vi "my_tracking.vi"() -> ()   [LabVIEW 2020]
uses:
  <vilib>/Utility/file.llb/Read Delimited Spreadsheet (DBL).vi
  <vilib>/Instr/_visa.llb/VISA Configure Serial Port (Instr).vi
panel:
  in  "VISA resource name":refnum<visa-resource-name>
  out "UTC":dbl
  out "Longtitude":dbl
  out "Latitude":dbl
  out "도(lat)":string
  out "도분초(lat)":string
  out "도(lon)":string
  out "도분초(lon)":string
  out "XYGraph":cluster{"array":dbl[], "array":dbl[]}[](graph)
  out "Satellited Used":string
  out "Fix Position":string
  out "velocity":dbl
  out "String":string
  out "error out":errorcluster
  out "XY graph":cluster{"X":dbl, "Y":dbl}[](graph)
  out "XY DATA":cluster{"X":dbl, "Y":dbl}[](array[cluster])
  out "Clustering graph":T1(graph)
  out "Safe Box Plotting":cluster{dbl[], dbl[]}[](graph)
  out "Box Point Array":cluster{dbl[], dbl[]}[](array[cluster])
  in  "?":enum32{"State", "ETC"}(tab)
  in  "stop":bool
  in  "file path (dialog if empty)":path caption="RDDF"
  out "XY Graph":T2(graph)
  in  "Refresh":bool
  in  "A/M":bool=TRUE
  in  "Serial Name":refnum<visa-resource-name>="COM8"
  out "ERP_Serial_DATA(RAW)":string
  in  "Vel":dbl=4.0 format="%#_13g"
  out "Index(near vehicle)":i32
  out "WP_no.":i32
  out "TM_Y":dbl format="%#_6f"
  out "TM_X":dbl format="%#_6f"
  out "True_Heading":dbl
  out "x_lat_path":dbl[](array[numeric])
  out "y_long_path":dbl[](array[numeric])
  out "vel. path":dbl[](array[numeric])
  out "Path_Vel_arr":dbl[](array[numeric])
  out "Path_long_arr":dbl[](array[numeric])
  out "Path_lat_arr":dbl[](array[numeric])
  out "ERP_Receive":T3
  out "Steer_CMD(Deg)":dbl
  out "CMD_2_ERP":T4
  out "Brake":u8
  out "Tracking_Error(m)":dbl
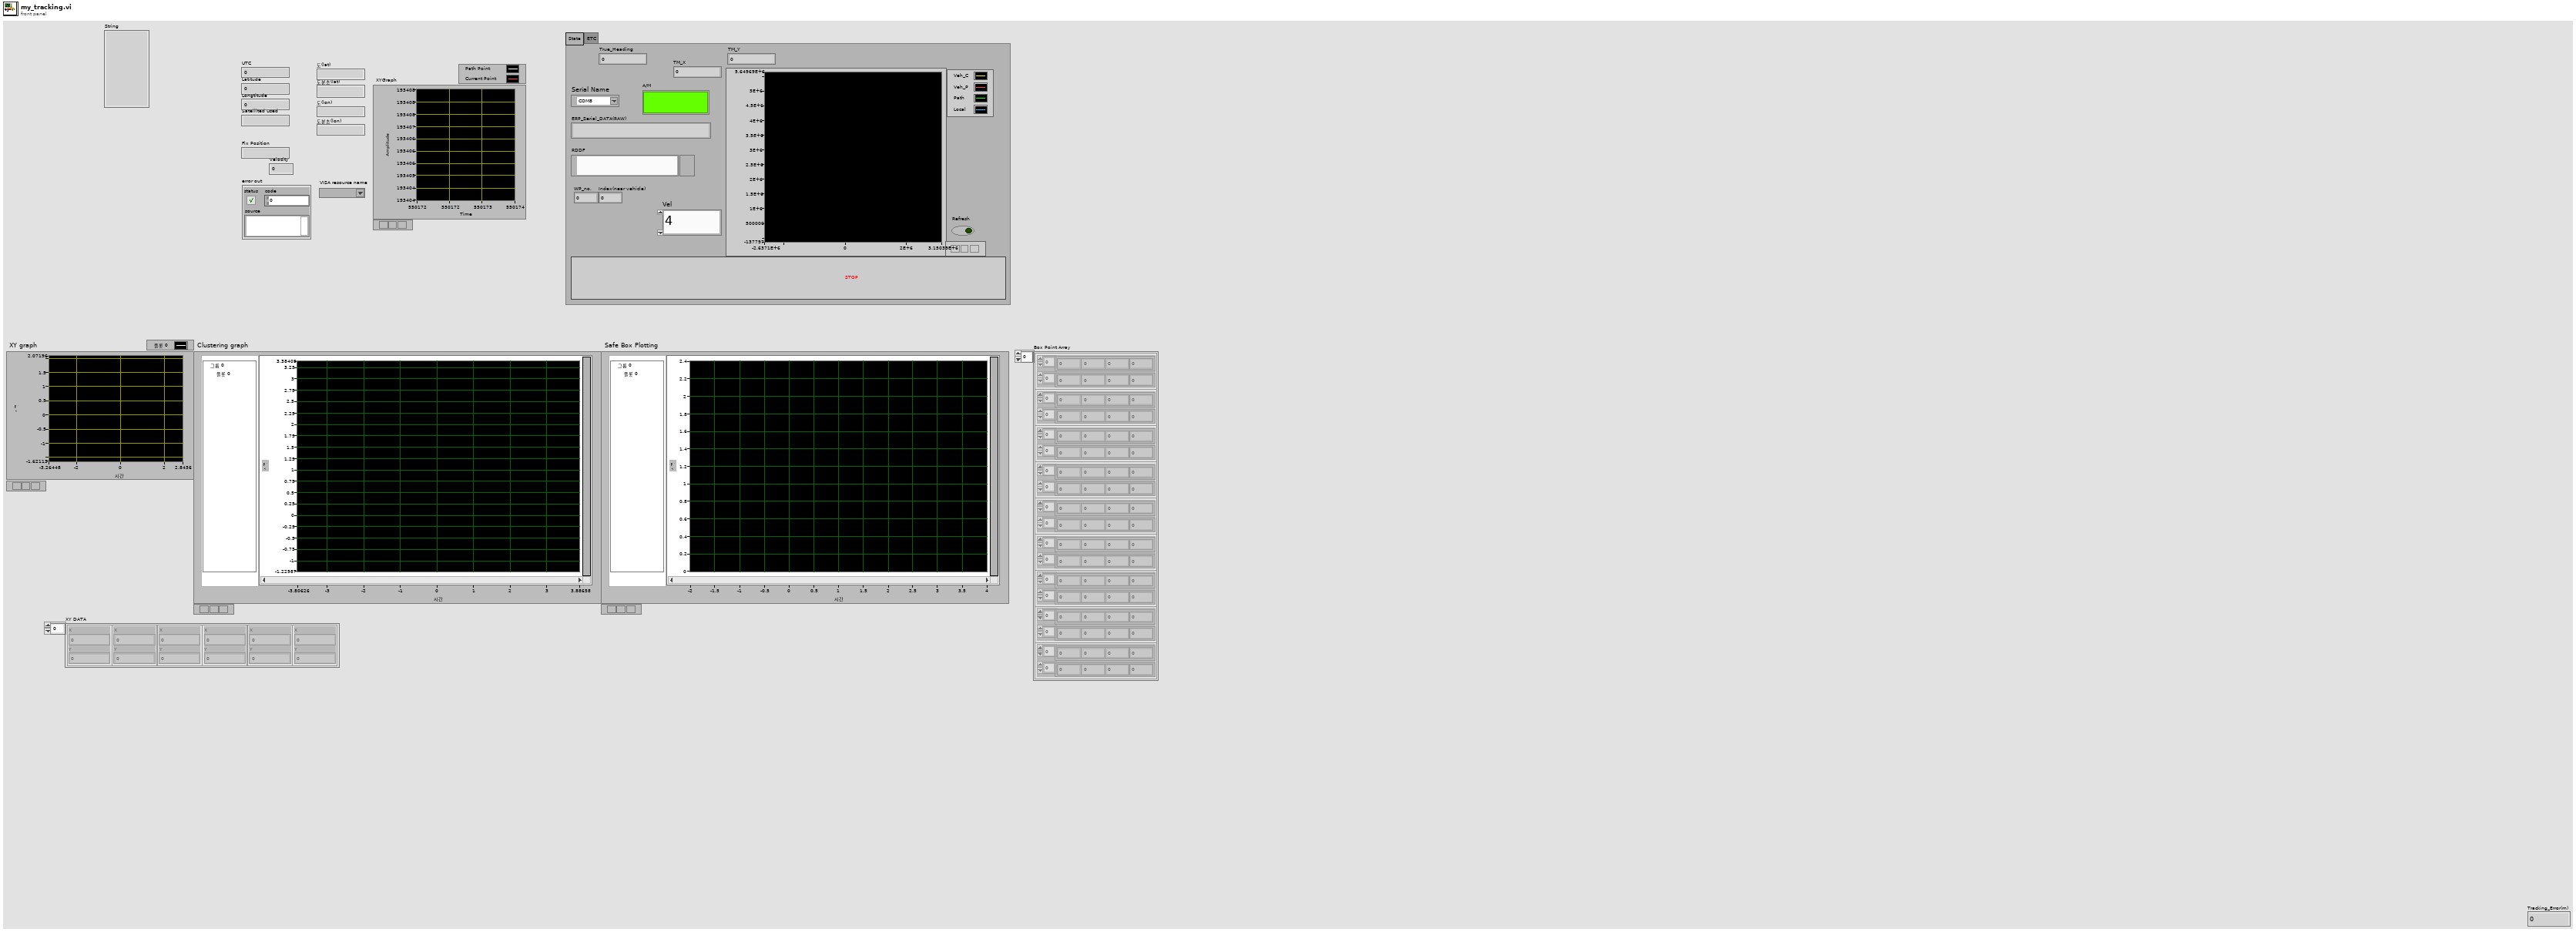
[diagram p1: front panel]
types:
  T1 = cluster{"최종 클러스터링 배열":cluster{"X":dbl, "Y":dbl}[]}[]
  T2 = cluster{"y_long_path":dbl[], "x_lat_path":dbl[]}[]
  T3 = cluster{"AorM":u8, "E-Stop":u8, "F_B":u8, "Speed":u16, "Steer":i16, "Brake":u8, "Encoder":u8, "Encoder 2":u8, "Encoder 3":u8, "Encoder 4":u8, "ALIVE":u8, "ETX_0":u8, "ETX_0 2":u8}
  T4 = cluster{"F/B":u8, "Speed":u16, "Steer":i16, "A/M":u8, "Brake":u8}
  T5 = cluster{"S":u8, "T":u8, "X":u8, "AorM":u8, "E-Stop":u8, "F_B":u8, "Speed":u16, "Steer":i16, "Brake":u8, "ALIVE":u8, "ETX_0":u8, "ETX_0 2":u8}
  T6 = cluster{"Path_long_arr":dbl[], "Path_lat_arr":dbl[]}
  T7 = cluster{"Path_long_arr":dbl[], "Path_lat_arr":dbl[]}[]
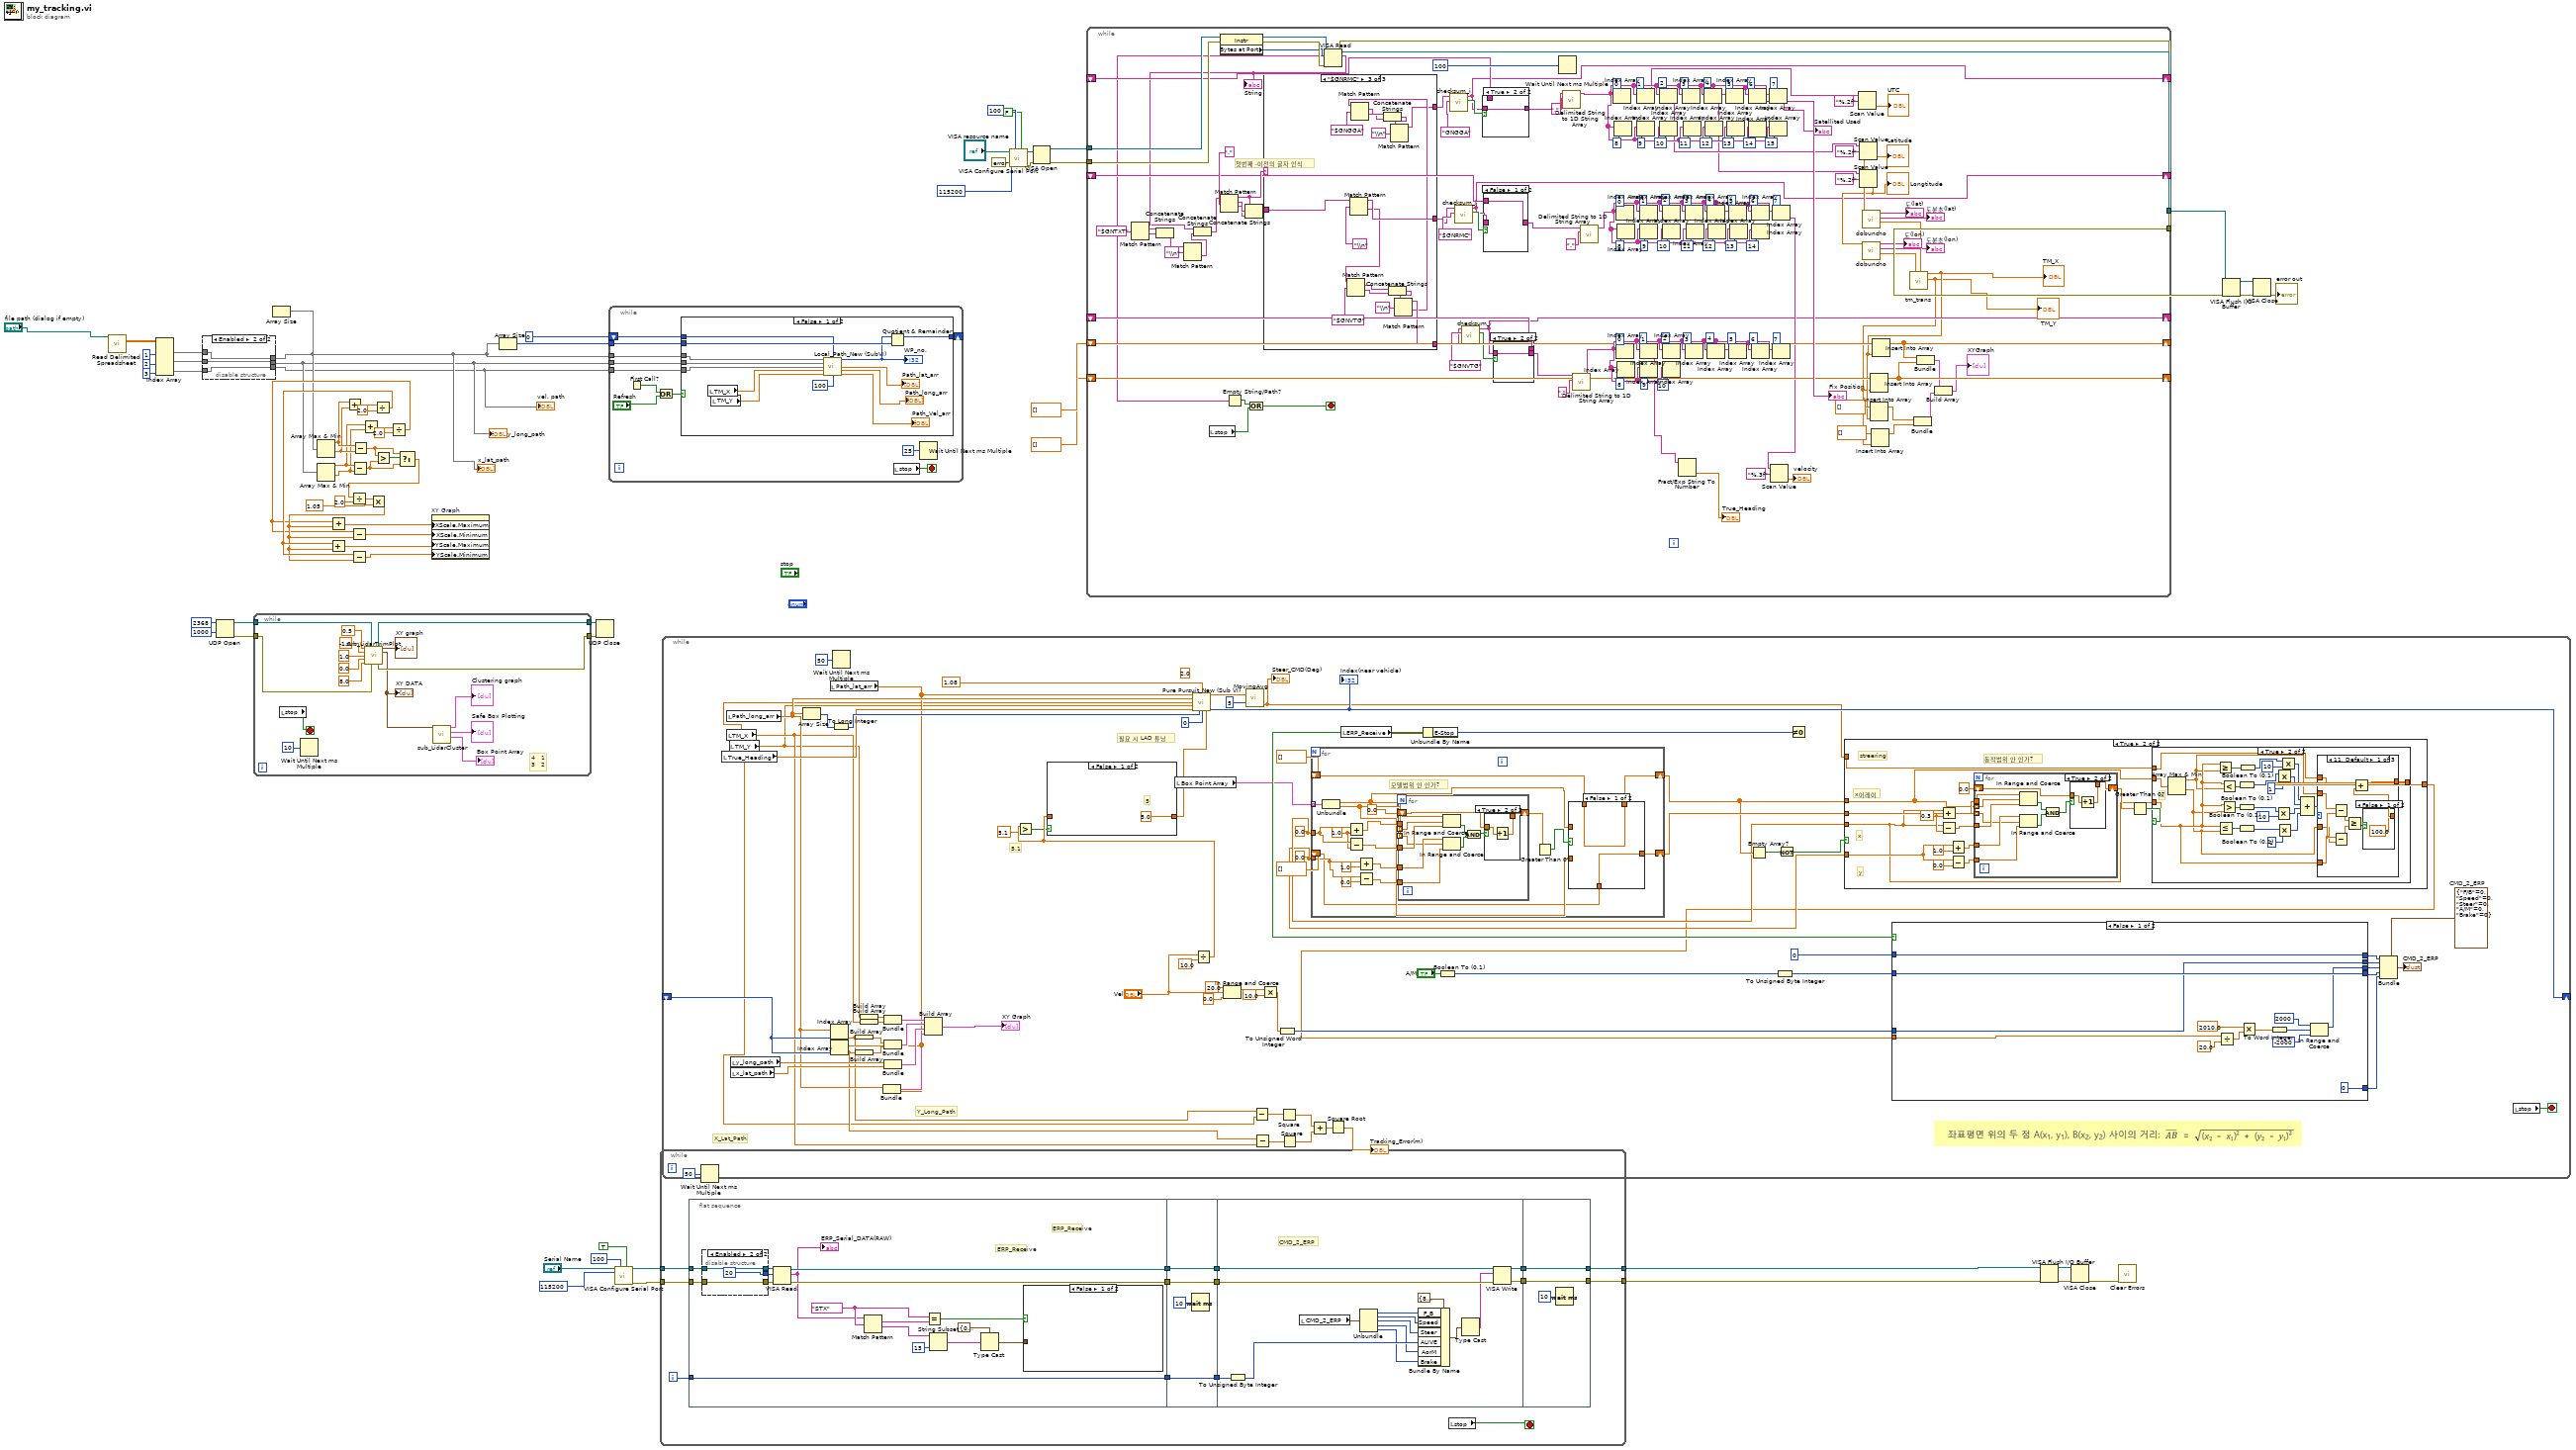
[diagram p0: block diagram]
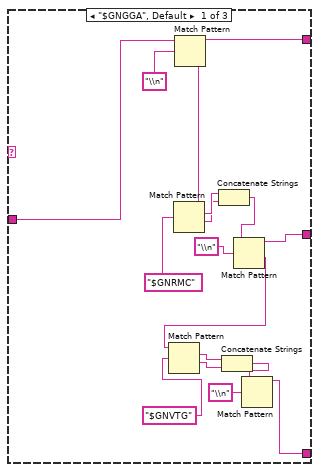
[diagram p5: hidden frame]
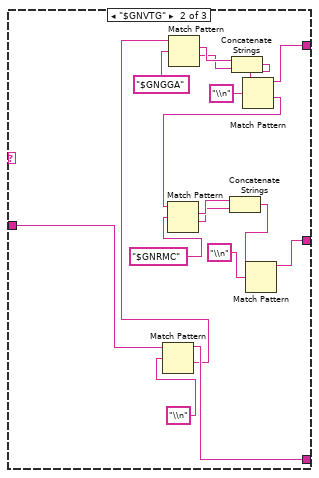
[diagram p6: hidden frame]
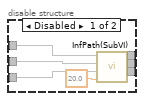
[diagram p7: hidden frame]
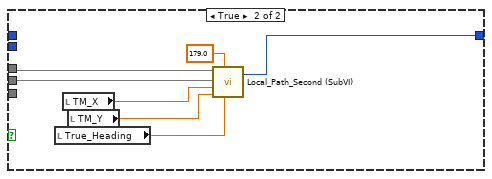
[diagram p8: hidden frame]
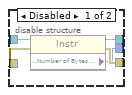
[diagram p9: hidden frame]
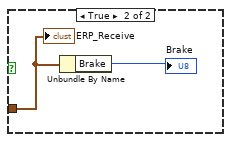
[diagram p10: hidden frame]
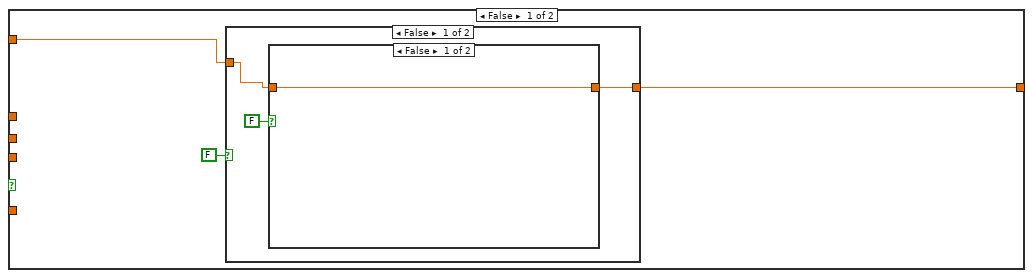
[diagram p11: hidden frame]
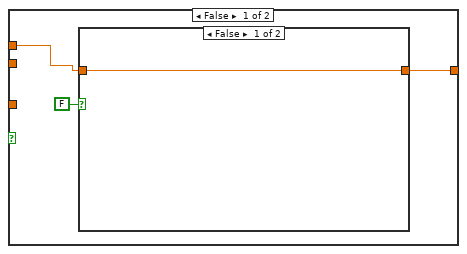
[diagram p15: hidden frame]
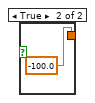
[diagram p17: hidden frame]
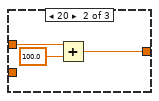
[diagram p18: hidden frame]
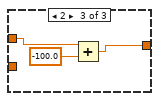
[diagram p19: hidden frame]
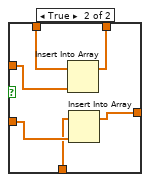
[diagram p20: hidden frame]
diagram:
  n1 = call-poly <vilib>:"Read Delimited Spreadsheet.vi"("file path (dialog if empty)"="file path (dialog if empty)") -> ("all rows"=w29:dbl[][])  [unwired: 9 in, 5 out]
  n2 = Index Array(array=w29, index (col) #1=1 ("비활성화된 인덱스 (열)"), index (col) #2=2 ("인덱스 (열)"), index (col) #3=3 ("인덱스 (열)")) -> (element #1=w54:dbl[], element #2=w53:dbl[], element #3=w52:dbl[])  [unwired: 3 in]
  n3 = disable-structure shown="Enabled" {
    disable-tunnel: w54 -> [w75 w78]
    disable-tunnel: w53 -> [w74 w77]
    disable-tunnel: w52 -> [w73 w76]
    disable-tunnel: [w72 w77] -> w18
    disable-tunnel: [w71 w76] -> w17
    disable-tunnel: [w70 w78] -> w19
    frame Disabled {
      n4 = call "InfPath(SubVI).vi"("Mod dist."=20.0, "vel."=w73, "y_long"=w74, "x_lat"=w75) -> ("vel. path"=w71:dbl[], "y_long_path"=w72:dbl[], "x_lat_path"=w70:dbl[])  [unwired: 1 out]
    }
    frame Enabled {
    }
  }
  "vel. path" <- w17
  "x_lat_path" <- w19
  "y_long_path" <- w18
  n5 = UDP Open(9:1000 ("타임아웃 ms (25000)"), 11:u16 2368 ("포트")) -> (port=w23:refnum<k16>, 0:w24:errorcluster)  [unwired: 3 in, 1 out]
  n6 = while {
    tunnel: w23 -> [w88]
    tunnel: w24 -> [w87]
    tunnel: [w86] -> w22
    tunnel: [w85] -> w21
    stop <- w79 stop-if-true
    # "4   1\n3   2"
    n7 = local read "stop"() -> (w79:bool)
    n8 = Wait Until Next ms Multiple(millisecond multiple=u32 10 ("ms 배수")) -> ()  [unwired: 1 out]
    n9 = call "sub_LidarTrimPlot.vi"("R_min"=0.5, "UDP 네트워크 연결 입력"=w88, "x-"=-1.0, "x+"=1.0, "y-"=0.0, "y+"=8.0, "에러 입력(에러 없음)"=w87) -> ("UDP 네트워크 연결 출력"=w86:refnum<k16>, "Point Cloud Plotting"=→"XY graph":cluster{"X":dbl, "Y":dbl}[], "trim XY DATA"=w83:cluster{"X":dbl, "Y":dbl}[], "에러 출력"=w85:errorcluster)  [unwired: 5 in]
    "XY DATA" <- w83
    n10 = call "sub_LidarCluster.vi"("XY DATA"=w83) -> ("Box Point Array"=→"Box Point Array":cluster{dbl[], dbl[]}[], "Safe Box Plotting"=→"Safe Box Plotting":cluster{dbl[], dbl[]}[], "Cluster Plotting"=→"Clustering graph":T1)  [unwired: 8 in]
  }
  n11 = Array Size(array=w19) -> ()  [unwired: 1 out]
  n12 = Array Max & Min(array=w18) -> (max value=w40:dbl, min value=w39:dbl)  [unwired: 2 out]
  n13 = Array Max & Min(array=w19) -> (max value=w46:dbl, min value=w45:dbl)  [unwired: 2 out]
  n14 = Add(x=w46, y=w45) -> (x+y=w43:dbl)
  n15 = Subtract(x=w40, y=w39) -> (x-y=w49:dbl)
  n16 = Subtract(x=w46, y=w45) -> (x-y=w50:dbl)
  n17 = Add(x=w40, y=w39) -> (x+y=w42:dbl)
  n18 = Divide(x=w43, y=2.0) -> (x/y=w36:dbl)
  n19 = Greater?(x=w50, y=w49) -> (0:w51:bool)
  n20 = Divide(x=w42, y=2.0) -> (x/y=w28:dbl)
  n21 = Select(t=w50, s=w51, f=w49) -> (s? t:f=w47:dbl)
  n22 = Divide(x=w47, y=2.0) -> (x/y=w38:dbl)
  n23 = Multiply(x=w38, y=1.05) -> (x*y=w35:dbl)
  n24 = Add(x=w36, y=w35) -> (x+y=w33:dbl)
  n25 = Add(x=w28, y=w35) -> (x+y=w31:dbl)
  n26 = Subtract(x=w28, y=w35) -> (x-y=w32:dbl)
  n27 = Subtract(x=w36, y=w35) -> (x-y=w34:dbl)
  n28 = property on="XY Graph" class="XYGraph (strict)"("XScale.Maximum"=w31, "XScale.Minimum"=w32, "YScale.Maximum"=w33, "YScale.Minimum"=w34) -> ()  [unwired: 2 in, 2 out]
  n29 = Array Size(array=w19) -> (size(s)=w30:i32)
  n30 = UDP Close(connection ID=w22, 8:w21) -> ()  [unwired: 2 out]
  n31 = while {
    tunnel: w19 -> [w104]
    tunnel: w18 -> [w103]
    tunnel: w17 -> [w101]
    tunnel: w30 -> [w100]
    shift-right: [w99] -> _
    shift-left: 0 ("Index0") -> [w102]
    stop <- w105 stop-if-true
    n32 = First Call?() -> (First Call?: T/F=w97:bool)
    n33 = Or(x=w97, y="Refresh") -> (x .or. y?=w98:bool)
    n34 = case shown="False" w98 {
      tunnel: w104 -> [w110 w125]
      tunnel: w103 -> [w112 w124]
      tunnel: w102 -> [w113 _]
      tunnel: w101 -> [w111 _]
      tunnel: w100 -> [w117 _]
      tunnel: [w118 w119] -> w99
      frame False {
        n35 = local read "TM_X"() -> (w116:dbl)
        n36 = local read "TM_Y"() -> (w115:dbl)
        n37 = call "Local_Path_New (SubVI).vi"("x_lat_arr"=w110, "WP no_pre"=w113, "y_long_arr"=w112, "vel_arr"=w111, "x_lat_c"=w116, "y_long_c"=w115, "# of pnt"=100) -> ("INDEX(Near Point)"=w107:i32, "Lat(Local)"=→"Path_lat_arr":dbl[], "Long(Local)"=→"Path_long_arr":dbl[], "Vel(Local)"=→"Path_Vel_arr":dbl[])  [unwired: 5 in]
        "WP_no." <- w107
        n38 = Quotient & Remainder(x=w107, y=w117) -> (x-y*floor(x/y)=w118:i32)  [unwired: 1 out]
      }
      frame True {
        n39 = local read "True_Heading"() -> (w121:dbl)
        n40 = local read "TM_X"() -> (w123:dbl)
        n41 = local read "TM_Y"() -> (w122:dbl)
        n42 = call "Local_Path_Second (SubVI).vi"("heading_deg"=w121, "heading_limit"=179.0, "y_long"=w122, "x_lat"=w123, "Y_long_path"=w124, "X_lat_path"=w125) -> ("Index(near vehicle)"=w119:i32)  [unwired: 1 out]
      }
    }
    n43 = local read "stop"() -> (w105:bool)
    n44 = Wait Until Next ms Multiple(millisecond multiple=u32 25) -> ()  [unwired: 1 out]
  }
  n45 = call-poly "VISA Configure Serial Port"("VISA resource name"="Serial Name", "timeout (10sec)"=u32 100, "Enable Termination\nChar (T)"=TRUE ("Enable Termination\nChar (T)"), "baud rate (9600)"=u32 115200) -> ("VISA resource name out"=w60:refnum<visa-resource-name>, "error out"=w59:errorcluster)  [unwired: 10 in]
  n46 = while {
    tunnel: w60 -> [w139]
    tunnel: w59 -> [w138]
    tunnel: [w136] -> w62
    tunnel: [w135] -> w61
    i -> [w137]
    stop <- w128 stop-if-true
    n47 = flat-sequence {
      tunnel: w139 -> [w157]
      tunnel: w138 -> [w156]
      tunnel: [w155] -> w134
      tunnel: [w154] -> w132
      tunnel: w137 -> [w153]
      tunnel: [w153] -> w130
      tunnel: w134 -> [w171]
      tunnel: [w171] -> w133
      tunnel: w132 -> [w170]
      tunnel: [w170] -> w131
      tunnel: w130 -> [w169]
      tunnel: [w169] -> w129
      tunnel: w133 -> [w184]
      tunnel: w131 -> [w183]
      tunnel: w129 -> [w181]
      tunnel: [w180] -> w127
      tunnel: [w179] -> w126
      tunnel: [w188] -> w135
      tunnel: [w189] -> w136
      tunnel: w127 -> [w189]
      tunnel: w126 -> [w188]
      frame #0 {
        w147 = "STX" ("검색 문자열/문자 (-)")
        # "ERP_Receive"
        # "ERP_Receive"
        n48 = disable-structure shown="Enabled" {
          disable-tunnel: w157 -> [w162 w164]
          disable-tunnel: w156 -> [w161 w165]
          disable-tunnel: [w160 w165] -> w152
          disable-tunnel: [w159 u32 20 ("timeout (10sec)")] -> w151
          disable-tunnel: [w158 w164] -> w150
          frame Disabled {
            n49 = property class="Instr"(reference=w162, error in=w161) -> (reference out=w158:refnum<visa-resource-name>, error out=w160:errorcluster, "Serial Settings:Number of Bytes at Serial Port"=w159:u32)
          }
          frame Enabled {
          }
        }
        n50 = VISA Read(VISA resource name=w150, byte count=w151, error in (no error)=w152) -> (VISA resource name out=w155:refnum<visa-resource-name>, read buffer=w145:string, error out=w154:errorcluster)  [unwired: 1 out]
        "ERP_Serial_DATA(RAW)" <- w145
        n51 = Match Pattern(string=w145, regular expression=w147) -> (match substring=w146:string, after substring=w149:string)  [unwired: 1 in, 2 out]
        n52 = Equal?(x=w147, y=w146) -> (x = y?=w144:bool)
        n53 = String Subset(string=w149, length (rest)=15 ("길이(나머지)")) -> (substring=w143:string)  [unwired: 1 in]
        n54 = Type Cast(type=T3 {"AorM"=0, "E-Stop"=0, "F_B"=0, "Speed"=0, "Steer"=0, "Brake"=0, "Encoder"=0, "Encoder 2"=0, "Encoder 3"=0, "Encoder 4"=0, "ALIVE"=0, "ETX_0"=13, "ETX_0 2"=10}, x=w143) -> (*(type *) &x=w142:T3)
        n55 = case shown="False" w144 {
          tunnel: w142 -> [_ w167]
          frame False {
          }
          frame True {
            n56 = Unbundle By Name(w167) -> ("Brake"=→"Brake":u8)
            "ERP_Receive" <- w167
          }
        }
      }
      frame #1 {
        n57 = Wait (ms)(milliseconds to wait=u32 10 ("대기 시간(ms)")) -> ()  [unwired: 1 out]
      }
      frame #2 {
        # "CMD_2_ERP"
        n58 = To Unsigned Byte Integer(number=w181) -> (unsigned 8bit integer=w186:u8)
        n59 = local read "CMD_2_ERP"() -> (w173:T4)
        n60 = Unbundle(w173) -> ("F/B"=w178:u8, "Speed"=w177:u16, "Steer"=w176:i16, "A/M"=w174:u8, "Brake"=w172:u8)
        n61 = Bundle By Name(cluster=T5 {"S"=83, "T"=84, "X"=88, "AorM"=0, "E-Stop"=0, "F_B"=0, "Speed"=0, "Steer"=0, "Brake"=0, "ALIVE"=0, "ETX_0"=13, "ETX_0 2"=10}, "F_B"=w178, "Speed"=w177, "Steer"=w176, "ALIVE"=w186, "AorM"=w174, "Brake"=w172) -> (w185:T5)
        n62 = Type Cast(x=w185) -> (*(type *) &x=w182:string)  [unwired: 1 in]
        n63 = VISA Write(VISA resource name=w184, write buffer=w182, error in (no error)=w183) -> (VISA resource name out=w180:refnum<visa-resource-name>, error out=w179:errorcluster)  [unwired: 1 out]
      }
      frame #3 {
        n64 = Wait (ms)(milliseconds to wait=u32 10 ("대기 시간(ms)")) -> ()  [unwired: 1 out]
      }
    }
    n65 = Wait Until Next ms Multiple(millisecond multiple=u32 50 ("ms 배수")) -> ()  [unwired: 1 out]
    n66 = local read "stop"() -> (w128:bool)
  }
  n67 = while {
    shift-right: [w247] -> _
    shift-left: _ -> [w244]
    stop <- w253 stop-if-true
    w192 = 0.0 ("TM_Y")
    w193 = 0.0 ("TM_X")
    w219 = T4 {"F/B"=0, "Speed"=0, "Steer"=0, "A/M"=0, "Brake"=0}  # CMD_2_ERP
    (unwired) 2.0 ("L")
    # "5.1"
    # "X_Lat_Path"
    # "Y_Long_Path"
    # "필요 시 LAD 튜닝"
    n68 = local read "True_Heading"() -> (w240:dbl)
    n69 = local read "Path_long_arr"() -> (w216:dbl[])
    n70 = local read "TM_X"() -> (w201:dbl)
    n71 = local read "TM_Y"() -> (w200:dbl)
    n72 = local read "y_long_path"() -> (w224:dbl[])
    n73 = local read "x_lat_path"() -> (w223:dbl[])
    n74 = Array Size(array=w216) -> (size(s)=w248:i32)
    n75 = local read "Path_lat_arr"() -> (w215:dbl[])
    n76 = Index Array(array=w216, index=w244) -> (element=w206:dbl)
    n77 = Index Array(array=w215, index=w244) -> (element=w205:dbl)
    n78 = Wait Until Next ms Multiple(millisecond multiple=u32 50 ("ms 배수")) -> ()  [unwired: 1 out]
    n79 = To Long Integer(number=w248) -> (32bit integer=w246:i32)
    n80 = Build Array(w206) -> (w255:dbl[])
    n81 = Build Array(w205) -> (w254:dbl[])
    n82 = Build Array(w200) -> (w257:dbl[])
    n83 = Build Array(w201) -> (w256:dbl[])
    n84 = Bundle("Path_long_arr"=w216, "Path_lat_arr"=w215) -> (w236:T6)  [unwired: 1 in]
    n85 = Bundle(w257, w256) -> (w242:cluster{dbl[], dbl[]})  [unwired: 1 in]
    n86 = Bundle(w255, w254) -> (w241:cluster{dbl[], dbl[]})  [unwired: 1 in]
    n87 = Bundle("y_long_path"=w224, "x_lat_path"=w223) -> (w243:cluster{"y_long_path":dbl[], "x_lat_path":dbl[]})  [unwired: 1 in]
    n88 = Build Array(w242, w241, w243, w236) -> (→"XY Graph":T7)
    n89 = local read "Box Point Array"() -> (w202:cluster{dbl[], dbl[]}[])
    n90 = Divide(x="Vel", y=10.0) -> (x/y=w237:dbl)
    n91 = Greater?(x=w237, y=5.1) -> (0:w204:bool)
    n92 = case shown="False" w204 {
      tunnel: w237 -> [_ w388]
      tunnel: [5.0 w387] -> w239
      frame False {
        # "5"
      }
      frame True {
        w389 = 3.7978021978021976  # intercept
        w391 = 0.23736263736263735  # slope
        n93 = Multiply(x=w391, y=w388) -> (x*y=w390:dbl)
        n94 = Add(x=w390, y=w389) -> (x+y=w387:dbl)
      }
    }
    n95 = call "Pure Pursuit_New (Sub VI).vi"("x_lat_path"=w215, "L"=1.08, "y_long_path"=w216, "X_Current"=w201, "Y_Current"=w200, "Heading_Current"=w240, "#pnt"=w246, "WP no_pre"=0, "LAD"=w239) -> ("Steer_CMD(Deg)"=w214:dbl, "Index(near vehicle)"=w247:i32)  [unwired: 5 in]
    "Index(near vehicle)" <- w247
    n96 = In Range and Coerce(upper limit=20.0 ("상위 리미트"), x="Vel", lower limit=0.0 ("하위 리미트")) -> (coerced(x)=w228:dbl)  [unwired: 1 out]
    n97 = call "MovingAvg.vi"("입력"=w214, "이동평균을 구할 자료의 개수"=u16 5) -> ("이동평균"=w191:dbl)  [unwired: 2 out]
    "Steer_CMD(Deg)" <- w191
    n98 = Subtract(x=w206, y=w200) -> (x-y=w211:dbl)
    n99 = Subtract(x=w205, y=w201) -> (x-y=w210:dbl)
    n100 = Multiply(x=w228, y=10.0) -> (x*y=w226:dbl)
    n101 = To Unsigned Word Integer(number=w226) -> (unsigned 16bit integer=w232:u16)
    n102 = Square(x=w211) -> (x^2=w209:dbl)
    n103 = Square(x=w210) -> (x^2=w208:dbl)
    n104 = for {
      tunnel: w202 -> [w363] mode=indexing
      tunnel: w193 -> [w356]
      tunnel: w192 -> [w354]
      shift-right: [w348] -> w196
      shift-left: dbl[] [] -> [w349]
      shift-right: [w346] -> w197
      shift-left: dbl[] [] -> [w345]
      w355 = 1.0 ("y")
      # "모델범위 안 인가?"
      n105 = Unbundle(w363) -> (w350:dbl[], w347:dbl[])
      n106 = Add(x=w356, y=w355) -> (x+y=w360:dbl)
      n107 = Subtract(x=w356, y=w355) -> (x-y=w359:dbl)
      n108 = Add(x=w354, y=1.0) -> (x+y=w358:dbl)
      n109 = Subtract(x=w354, y=0.0) -> (x-y=w357:dbl)
      n110 = for {
        tunnel: w350 -> [w380] mode=indexing
        tunnel: w347 -> [w377] mode=indexing
        tunnel: w360 -> [w382]
        tunnel: w359 -> [w381]
        tunnel: w358 -> [w379]
        tunnel: w357 -> [w378]
        shift-right: [w372] -> w353
        shift-left: 0.0 -> [w373]
        n111 = In Range and Coerce(upper limit=w382, x=w380, lower limit=w381) -> (In Range?=w376:bool)  [unwired: 1 out]
        n112 = In Range and Coerce(upper limit=w379, x=w377, lower limit=w378) -> (In Range?=w375:bool)  [unwired: 1 out]
        n113 = And(x=w376, y=w375) -> (x .and. y?=w374:bool)
        n114 = case shown="True" w374 {
          tunnel: w373 -> [w383 w385]
          tunnel: [w383 w384] -> w372
          frame False {
          }
          frame True {
            n115 = Increment(x=w385) -> (x+1=w384:dbl)
          }
        }
      }
      n116 = Greater Than 0?(x=w353) -> (x > 0?=w351:bool)
      n117 = case shown="False" w351 {
        tunnel: w350 -> [_ w371]
        tunnel: w349 -> [w365 w370]
        tunnel: [w365 w369] -> w348
        tunnel: w347 -> [_ w368]
        tunnel: [w364 w367] -> w346
        tunnel: w345 -> [w364 w366]
        frame False {
        }
        frame True {
          n118 = Insert Into Array(array=w370, new element=w371) -> (w369:dbl[])  [unwired: 1 in]
          n119 = Insert Into Array(array=w366, new element=w368) -> (w367:dbl[])  [unwired: 1 in]
        }
      }
    }
    n120 = Add(x=w209, y=w208) -> (x+y=w207:dbl)
    n121 = Square Root(x=w207) -> (sqrt(x)=→"Tracking_Error(m)":dbl)
    n122 = local read "ERP_Receive"() -> (w250:T3)
    n123 = Unbundle By Name(w250) -> ("E-Stop"=w251:u8)
    n124 = Boolean To (0,1)(Boolean="A/M") -> (0, 1=w235:i16)
    n125 = Empty Array?(array=w196) -> (empty?=w195:bool)
    n126 = To Unsigned Byte Integer(number=w235) -> (unsigned 8bit integer=w217:u8)
    n127 = Not(x=w195) -> (.not. x?=w194:bool)
    n128 = Not Equal To 0?(x=w251) -> (x != 0?=w231:bool)
    n129 = case shown="True" w194 {
      tunnel: w191 -> [w263 w285]
      tunnel: [w262 w284] -> w190
      tunnel: w196 -> [_ w270]
      tunnel: w197 -> [_ w283]
      tunnel: w193 -> [_ w271]
      tunnel: w192 -> [_ w279]
      frame False {
        n130 = case shown="False" FALSE {
          tunnel: w263 -> [w266 w269]
          tunnel: [w265 w269] -> w262
          frame False {
            n131 = case shown="False" FALSE {
              tunnel: w266 -> [w267 w268]
              tunnel: [w267 w268] -> w265
              frame False {
              }
              frame True {
              }
            }
          }
          frame True {
          }
        }
      }
      frame True {
        w280 = 0.3 ("y")
        # "y"
        # "x"
        # "streering"
        # "x어레이"
        # "동작범위 안 인가?"
        n132 = Add(x=w271, y=w280) -> (x+y=w278:dbl)
        n133 = Subtract(x=w271, y=w280) -> (x-y=w277:dbl)
        n134 = Add(x=w279, y=1.0) -> (x+y=w276:dbl)
        n135 = Subtract(x=w279, y=0.0) -> (x-y=w275:dbl)
        n136 = for {
          tunnel: w270 -> [w294] mode=indexing
          tunnel: w283 -> [w291] mode=indexing
          tunnel: w278 -> [w296]
          tunnel: w277 -> [w295]
          tunnel: w276 -> [w293]
          tunnel: w275 -> [w292]
          shift-right: [w288] -> w273
          shift-left: 0.0 -> [w287]
          n137 = In Range and Coerce(upper limit=w296, x=w294, lower limit=w295) -> (In Range?=w290:bool)  [unwired: 1 out]
          n138 = In Range and Coerce(upper limit=w293, x=w291, lower limit=w292) -> (In Range?=w289:bool)  [unwired: 1 out]
          n139 = And(x=w290, y=w289) -> (x .and. y?=w286:bool)
          n140 = case shown="True" w286 {
            tunnel: w287 -> [w297 w299]
            tunnel: [w297 w298] -> w288
            frame False {
            }
            frame True {
              n141 = Increment(x=w299) -> (x+1=w298:dbl)
            }
          }
        }
        n142 = Greater Than 0?(x=w273) -> (x > 0?=w272:bool)
        n143 = case shown="True" w272 {
          tunnel: w285 -> [w302 w310]
          tunnel: [w301 w309] -> w284
          tunnel: w271 -> [_ w308]
          tunnel: w270 -> [_ w307]
          frame False {
            n144 = case shown="False" FALSE {
              tunnel: w302 -> [w303 w304]
              tunnel: [w303 w304] -> w301
              frame False {
              }
              frame True {
              }
            }
          }
          frame True {
            # "x"
            n145 = Array Max & Min(array=w307) -> (max value=w306:dbl, min value=w305:dbl)  [unwired: 2 out]
            n146 = Greater Or Equal?(x=w308, y=w306) -> (x >= y?=w327:bool)
            n147 = Less Or Equal?(x=w308, y=w305) -> (x <= y?=w326:bool)
            n148 = Less?(x=w308, y=w306) -> (x < y?=w312:bool)
            n149 = Greater?(x=w308, y=w305) -> (0:w311:bool)
            n150 = Boolean To (0,1)(Boolean=w312) -> (0, 1=w319:i16)
            n151 = Boolean To (0,1)(Boolean=w311) -> (0, 1=w321:i16)
            n152 = Boolean To (0,1)(Boolean=w326) -> (0, 1=w320:i16)
            n153 = Boolean To (0,1)(Boolean=w327) -> (0, 1=w318:i16)
            n154 = Multiply(x=w321, y=i16 10) -> (x*y=w315:i16)
            n155 = Multiply(x=w319, y=i16 1) -> (x*y=w316:i16)
            n156 = Multiply(x=w320, y=i16 1) -> (x*y=w314:i16)
            n157 = Multiply(x=w318, y=i16 10) -> (x*y=w317:i16)
            n158 = Compound Arithmetic op=ADD(w317, w316, w315, w314) -> (w313:i16)
            n159 = case shown="11, Default" w313 {
              tunnel: w310 -> [w330 w341 w342]
              tunnel: [w328 w339 w343] -> w309
              tunnel: w306 -> [w335 _ _]
              tunnel: w305 -> [w334 _ _]
              tunnel: w308 -> [w336 _ _]
              frame 11, Default {
                n160 = Subtract(x=w335, y=w336) -> (x-y=w333:dbl)
                n161 = Subtract(x=w336, y=w334) -> (x-y=w332:dbl)
                n162 = Greater Or Equal?(x=w333, y=w332) -> (x >= y?=w331:bool)
                n163 = case shown="False" w331 {
                  tunnel: [100.0 -100.0] -> w329
                  frame False {
                  }
                  frame True {
                  }
                }
                n164 = Add(x=w330, y=w329) -> (x+y=w328:dbl)
              }
              frame 20 {
                n165 = Add(x=w341, y=100.0) -> (x+y=w339:dbl)
              }
              frame 2 {
                n166 = Add(x=w342, y=-100.0) -> (x+y=w343:dbl)
              }
            }
          }
        }
      }
    }
    n167 = case shown="False" w231 {
      tunnel: u8 0 -> [w404 _]
      tunnel: [w404 w406] -> w260
      tunnel: [w401 w406] -> w259
      tunnel: [w393 w406] -> w258
      tunnel: [w403 w406] -> w234
      tunnel: w217 -> [w403 _]
      tunnel: w190 -> [w402 _]
      tunnel: w232 -> [w401 _]
      tunnel: [u8 0 u8 200] -> w220
      frame False {
        n168 = Divide(x=w402, y=20.0) -> (x/y=w399:dbl)
        n169 = Multiply(x=2010.0, y=w399) -> (x*y=w398:dbl)
        n170 = To Word Integer(number=w398) -> (16bit integer=w400:i16)
        n171 = In Range and Coerce(upper limit=i16 2000 ("상위 리미트"), x=w400, lower limit=i16 -2000 ("하위 리미트")) -> (coerced(x)=w393:i16)  [unwired: 1 out]
      }
      frame True {
        w406 = u8 0
      }
    }
    n172 = Bundle(cluster=w219, "F/B"=w260, "Speed"=w259, "Steer"=w258, "A/M"=w234, "Brake"=w220) -> (→"CMD_2_ERP":T4)
    n173 = local read "stop"() -> (w253:bool)
  }
  n174 = call-poly "VISA Configure Serial Port"("VISA resource name"="VISA resource name", "timeout (10sec)"=u32 100, "Enable Termination\nChar (T)"=FALSE ("Enable Termination\nChar (T)"), "baud rate (9600)"=u32 115200 ("baud rate (115200)"), "error in (no error)"=errorcluster {"status"=FALSE, "code"=0, "source"=""}) -> ("VISA resource name out"=w6:refnum<visa-resource-name>, "error out"=w7:errorcluster)  [unwired: 9 in]
  n175 = VISA Open(error in (no error)=w7, VISA resource name=w6) -> (VISA resource name=w5:refnum<visa-resource-name>, error out=w4:errorcluster)  [unwired: 3 in]
  n176 = while {
    tunnel: w5 -> [w481]
    tunnel: w4 -> [w480]
    tunnel: [w470] -> w16
    tunnel: [w469] -> w15
    shift-right: [w432] -> _
    shift-left: _ -> [w452]
    shift-right: [w428] -> _
    shift-left: _ -> [w450]
    shift-right: [w425] -> _
    shift-left: _ -> [w448]
    shift-right: [w446] -> _
    shift-left: dbl[] [] -> [w447]
    shift-right: [w444] -> _
    shift-left: dbl[] [] -> [w445]
    stop <- w530 stop-if-true
    # "첫번째 ,이전의 글자 인식"
    n177 = local read "stop"() -> (w422:bool)
    n178 = property class="Instr"(reference=w481, error in=w480) -> (reference out=w479:refnum<visa-resource-name>, error out=w478:errorcluster, "Bytes at Port"=w468:u32)
    n179 = VISA Read(VISA resource name=w479, byte count=w468, error in (no error)=w478) -> (VISA resource name out=w470:refnum<visa-resource-name>, read buffer=w418:string, error out=w469:errorcluster)  [unwired: 1 out]
    n180 = Match Pattern(string=w418, regular expression="$GNTXT") -> (before substring=w412:string, match substring=w416:string, after substring=w415:string)  [unwired: 1 in, 1 out]
    n181 = Concatenate Strings(w416, w415) -> (w414:string)
    n182 = Match Pattern(string=w414, regular expression="\\n") -> (after substring=w411:string)  [unwired: 1 in, 3 out]
    n183 = Concatenate Strings(w412, w411) -> (w410:string)
    n184 = Match Pattern(string=w410, regular expression=",") -> (before substring=w462:string, match substring=w461:string, after substring=w460:string)  [unwired: 1 in, 1 out]
    n185 = Empty String/Path?(string/path=w418) -> (empty?=w531:bool)
    n186 = Concatenate Strings(w462, w461, w460) -> (w463:string)
    n187 = Or(x=w531, y=w422) -> (x .or. y?=w530:bool)
    n188 = case shown="\"$GNRMC\"" w462 {
      tunnel: w463 -> [w554 w571 w586]
      tunnel: [w546 w556 w585] -> w430
      tunnel: [w539 w569 w579] -> w426
      tunnel: [w553 w563 w573] -> w419
      frame "$GNGGA", Default {
        n189 = Match Pattern(string=w554, regular expression="\\n") -> (before substring=w553:string, after substring=w552:string)  [unwired: 1 in, 2 out]
        n190 = Match Pattern(string=w552, regular expression="$GNRMC") -> (match substring=w549:string, after substring=w548:string)  [unwired: 1 in, 2 out]
        n191 = Concatenate Strings(w549, w548) -> (w547:string)
        n192 = Match Pattern(string=w547, regular expression="\\n") -> (before substring=w546:string, after substring=w543:string)  [unwired: 1 in, 2 out]
        n193 = Match Pattern(string=w543, regular expression="$GNVTG") -> (match substring=w541:string, after substring=w540:string)  [unwired: 1 in, 2 out]
        n194 = Concatenate Strings(w541, w540) -> (w544:string)
        n195 = Match Pattern(string=w544, regular expression="\\n") -> (before substring=w539:string)  [unwired: 1 in, 3 out]
      }
      frame "$GNVTG" {
        n196 = Match Pattern(string=w571, regular expression="\\n") -> (before substring=w569:string, after substring=w568:string)  [unwired: 1 in, 2 out]
        n197 = Match Pattern(string=w568, regular expression="$GNGGA") -> (match substring=w565:string, after substring=w564:string)  [unwired: 1 in, 2 out]
        n198 = Concatenate Strings(w565, w564) -> (w566:string)
        n199 = Match Pattern(string=w566, regular expression="\\n") -> (before substring=w563:string, after substring=w562:string)  [unwired: 1 in, 2 out]
        n200 = Match Pattern(string=w562, regular expression="$GNRMC") -> (match substring=w558:string, after substring=w557:string)  [unwired: 1 in, 2 out]
        n201 = Concatenate Strings(w558, w557) -> (w559:string)
        n202 = Match Pattern(string=w559, regular expression="\\n") -> (before substring=w556:string)  [unwired: 1 in, 3 out]
      }
      frame "$GNRMC" {
        n203 = Match Pattern(string=w586, regular expression="\\n") -> (before substring=w585:string, after substring=w584:string)  [unwired: 1 in, 2 out]
        n204 = Match Pattern(string=w584, regular expression="$GNVTG") -> (match substring=w580:string, after substring=w581:string)  [unwired: 1 in, 2 out]
        n205 = Concatenate Strings(w580, w581) -> (w582:string)
        n206 = Match Pattern(string=w582, regular expression="\\n") -> (before substring=w579:string, after substring=w578:string)  [unwired: 1 in, 2 out]
        n207 = Match Pattern(string=w578, regular expression="$GNGGA") -> (match substring=w575:string, after substring=w574:string)  [unwired: 1 in, 2 out]
        n208 = Concatenate Strings(w575, w574) -> (w576:string)
        n209 = Match Pattern(string=w576, regular expression="\\n") -> (before substring=w573:string)  [unwired: 1 in, 3 out]
      }
    }
    n210 = call "checksum_i.vi"("check dataName"="GNGGA", "string"=w419) -> ("Boolean"=w433:bool, "String"=w432:string)  [unwired: 8 in]
    n211 = call "checksum_i.vi"("check dataName"="$GNRMC", "string"=w430) -> ("Boolean"=w429:bool, "String"=w428:string)  [unwired: 8 in]
    n212 = call "checksum_i.vi"("check dataName"="$GNVTG", "string"=w426) -> ("Boolean"=w424:bool, "String"=w425:string)  [unwired: 8 in]
    n213 = case shown="True" w433 {
      tunnel: [w537 w538] -> w453
      tunnel: w432 -> [_ w538]
      tunnel: w452 -> [w537 _]
      frame False {
      }
      frame True {
      }
    }
    n214 = case shown="False" w429 {
      tunnel: w428 -> [_ w536]
      tunnel: [w535 w536] -> w451
      tunnel: w450 -> [w535 _]
      frame False {
      }
      frame True {
      }
    }
    n215 = case shown="True" w424 {
      tunnel: w425 -> [_ w534]
      tunnel: [w533 w534] -> w449
      tunnel: w448 -> [w533 _]
      frame False {
      }
      frame True {
      }
    }
    n216 = Wait Until Next ms Multiple(millisecond multiple=u32 100) -> ()  [unwired: 1 out]
    n217 = call <vilib>:"Delimited String to 1D String Array.vi"("delimiter"=",", "delimited string"=w453) -> ("string array"=w529:string[])  [unwired: 9 in]
    n218 = call <vilib>:"Delimited String to 1D String Array.vi"("delimiter"=",", "delimited string"=w449) -> ("string array"=w494:string[])  [unwired: 9 in]
    n219 = call <vilib>:"Delimited String to 1D String Array.vi"("delimiter"=",", "delimited string"=w451) -> ("string array"=w511:string[])  [unwired: 9 in]
    n220 = Index Array(array=w529, index=0) -> ()  [unwired: 1 out]
    n221 = Index Array(array=w529, index=8) -> ()  [unwired: 1 out]
    n222 = Index Array(array=w511, index=0) -> ()  [unwired: 1 out]
    n223 = Index Array(array=w494, index=0) -> ()  [unwired: 1 out]
    n224 = Index Array(array=w511, index=8) -> ()  [unwired: 1 out]
    n225 = Index Array(array=w494, index=8) -> ()  [unwired: 1 out]
    n226 = Index Array(array=w529, index=1) -> (element=w475:string)
    n227 = Index Array(array=w529, index=9) -> ()  [unwired: 1 out]
    n228 = Index Array(array=w511, index=1) -> ()  [unwired: 1 out]
    n229 = Index Array(array=w511, index=9) -> ()  [unwired: 1 out]
    n230 = Index Array(array=w494, index=1) -> (element=w421:string)
    n231 = Index Array(array=w494, index=9) -> ()  [unwired: 1 out]
    n232 = Index Array(array=w529, index=2) -> (element=w472:string)
    n233 = Index Array(array=w529, index=10) -> ()  [unwired: 1 out]
    n234 = Index Array(array=w511, index=2) -> ()  [unwired: 1 out]
    n235 = Index Array(array=w511, index=10) -> ()  [unwired: 1 out]
    n236 = Index Array(array=w494, index=2) -> ()  [unwired: 1 out]
    n237 = Index Array(array=w494, index=10) -> ()  [unwired: 1 out]
    n238 = Fract/Exp String To Number(string=w421) -> (number=→"True_Heading":dbl)  [unwired: 3 in, 1 out]
    n239 = Index Array(array=w529, index=3) -> ()  [unwired: 1 out]
    n240 = Index Array(array=w529, index=11) -> ()  [unwired: 1 out]
    n241 = Index Array(array=w511, index=3) -> ()  [unwired: 1 out]
    n242 = Index Array(array=w494, index=3) -> ()  [unwired: 1 out]
    n243 = Index Array(array=w511, index=11) -> ()  [unwired: 1 out]
    n244 = Index Array(array=w529, index=4) -> (element=w471:string)
    n245 = Index Array(array=w529, index=12) -> ()  [unwired: 1 out]
    n246 = Index Array(array=w511, index=4) -> ()  [unwired: 1 out]
    n247 = Index Array(array=w494, index=4) -> ()  [unwired: 1 out]
    n248 = Index Array(array=w511, index=12) -> ()  [unwired: 1 out]
    n249 = Index Array(array=w529, index=5) -> ()  [unwired: 1 out]
    n250 = Index Array(array=w529, index=13) -> ()  [unwired: 1 out]
    n251 = Index Array(array=w511, index=5) -> ()  [unwired: 1 out]
    n252 = Index Array(array=w494, index=5) -> ()  [unwired: 1 out]
    n253 = Index Array(array=w511, index=13) -> ()  [unwired: 1 out]
    n254 = Index Array(array=w529, index=6) -> (element=→"Fix Position":string)
    n255 = Index Array(array=w529, index=14) -> ()  [unwired: 1 out]
    n256 = Index Array(array=w511, index=6) -> ()  [unwired: 1 out]
    n257 = Index Array(array=w494, index=6) -> ()  [unwired: 1 out]
    n258 = Index Array(array=w511, index=14) -> ()  [unwired: 1 out]
    n259 = Index Array(array=w529, index=7) -> (element=→"Satellited Used":string)
    n260 = Index Array(array=w529, index=15) -> ()  [unwired: 1 out]
    n261 = Index Array(array=w511, index=7) -> (element=w436:string)
    n262 = Scan Value(string=w436, format string="%.3f") -> (value=→"velocity":dbl)  [unwired: 1 in, 1 out]
    n263 = Index Array(array=w494, index=7) -> ()  [unwired: 1 out]
    n264 = Scan Value(string=w475, format string="%.2f") -> (value=→"UTC":dbl)  [unwired: 1 in, 1 out]
    n265 = Scan Value(string=w472, format string="%.2f") -> (value=w458:dbl)  [unwired: 1 in, 1 out]
    "Latitude" <- w458
    n266 = Scan Value(string=w471, format string="%.2f") -> (value=w457:dbl)  [unwired: 1 in, 1 out]
    "Longtitude" <- w457
    n267 = call "dobuncho.vi"("Numeric in"=w458) -> ("Numeric out"=w459:dbl, "String"=→"도분초(lat)":string, "String 2"=→"도(lat)":string)  [unwired: 8 in]
    n268 = call "dobuncho.vi"("Numeric in"=w457) -> ("Numeric out"=w454:dbl, "String"=→"도분초(lon)":string, "String 2"=→"도(lon)":string)  [unwired: 8 in]
    n269 = call "tm_trans.vi"("Long"=w454, "Lat"=w459) -> ("Numeric"=w407:dbl, "out_pt"=w408:dbl)  [unwired: 8 in]
    "TM_Y" <- w407
    "TM_X" <- w408
    n270 = Insert Into Array(array=w445, new element=w407) -> (w444:dbl[])  [unwired: 1 in]
    n271 = Insert Into Array(array=dbl[] [], new element=w408) -> (w441:dbl[])  [unwired: 1 in]
    n272 = Insert Into Array(array=dbl[] [], new element=w407) -> (w440:dbl[])  [unwired: 1 in]
    n273 = Insert Into Array(array=w447, new element=w408) -> (w446:dbl[])  [unwired: 1 in]
    n274 = Bundle("array"=w441, "array"=w440) -> (w439:cluster{"array":dbl[], "array":dbl[]})  [unwired: 1 in]
    n275 = Bundle(w446, w444) -> (w438:cluster{dbl[], dbl[]})  [unwired: 1 in]
    n276 = Build Array(w438, w439) -> (→"XYGraph":cluster{"array":dbl[], "array":dbl[]}[])
    "String" <- w452
  }
  n277 = VISA Flush I/O Buffer(VISA resource name=w62, error in (no error)=w61) -> (VISA resource name out=w63:refnum<visa-resource-name>, error out=w64:errorcluster)  [unwired: 1 in]
  n278 = VISA Close(VISA resource name=w63, error in (no error)=w64) -> (error out=w58:errorcluster)
  n279 = call <vilib>:"Clear Errors.vi"("error in (no error)"=w58) -> ()  [unwired: 5 in, 2 out]
  n280 = VISA Flush I/O Buffer(VISA resource name=w16, error in (no error)=w15) -> (VISA resource name out=w13:refnum<visa-resource-name>, error out=w14:errorcluster)  [unwired: 1 in]
  n281 = VISA Close(VISA resource name=w13, error in (no error)=w14) -> (error out=→"error out":errorcluster)
